vi "lut.vi"(1 "SOC":dbl[](array[numeric]), 2 "soc":dbl, 3 "param":dbl[](array[numeric])=[0.0, 10.0, 20.0, 30.0, 40.0, 50.0, 60.0, 70.0, 80.0, 90.0, 100.0]) -> (0 "param(soc)":dbl)   [LabVIEW 2021]
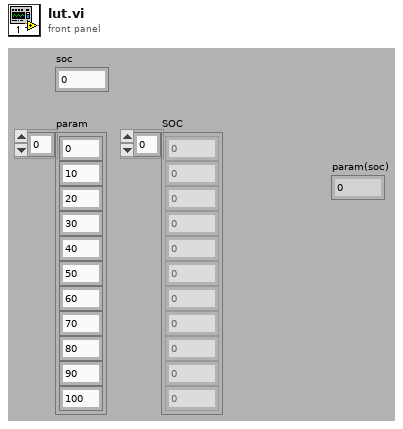
[diagram p1: front panel]
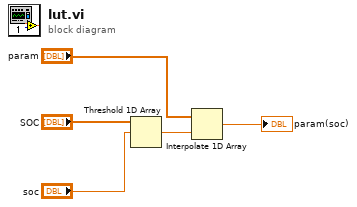
[diagram p0: block diagram]
diagram:
  n1 = Threshold 1D Array(2:"soc", 3:"SOC") -> (0:w4:dbl)  [unwired: 1 in]
  n2 = Interpolate 1D Array(1:w4, 2:"param") -> (0:→"param(soc)":dbl)
